vi "_CallDirectly.vi"() -> ()   [LabVIEW 2019, in "lv-providershell-example3.lvlib"]
uses:
  lv-providershell-example3.lvlib
  content/ContentClass.lvclass
panel:
  out "valid":bool
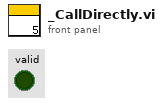
[diagram p1: front panel]
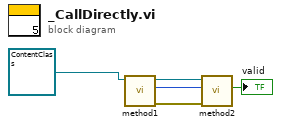
[diagram p0: block diagram]
diagram:
  n1 = call-dynamic "method1.vi"("ContentClass in"=refnum<class "ContentClass.lvclass"> refnum ("lv-providershell-example3.lvlib:ContentClass.lvclass")) -> ("error out"=w3:errorcluster, "RefNum"=w4:i32, "ContentClass out"=w5:refnum<class "ContentClass.lvclass">)  [unwired: 8 in]
  n2 = call-dynamic "method2.vi"("error in (no error)"=w3, "RefNum"=w4, "ContentClass in"=w5) -> ("Boolean"=→"valid":bool)  [unwired: 6 in, 2 out]
